vi "Connect.vi"(8 "error in (no error)":errorcluster, 9 "Custom Config Data":u8[](array[numeric]) format="%.0x", 10 "Connection Name":string, 11 "CIFTag in":refnum<class "CIF_NIChn.lvclass">) -> (0 "error out":errorcluster, 3 "CIFTag out":refnum<class "CIF_NIChn.lvclass">)   [LabVIEW 2021, in "CIF_NIChn.lvclass"]
uses:
  CIF_NIChn.lvclass
  D:/dev/CIF-LVCore/src/Channels/CIFChannels/CIFChannels.lvclass
  CIFChannels/CIFChannels.lvclass/CIFChannels.ctl
  CIFChannels/Typedef/Channel State.ctl
  CIFChannels/Accessors/Read Direction.vi
  CIFChannels/Accessors/Read Name.vi
  CIF_NIChn.lvclass/CIF_NIChn.ctl
  CIFChannels/CIFChannels.lvclass
  <vilib>/CIFChannels/CIFChannelCore.lvlib
  D:/dev/CIF-LVCore/src/Channels/CIF_NIChn/NIChn/CIF_NIChn.lvclass
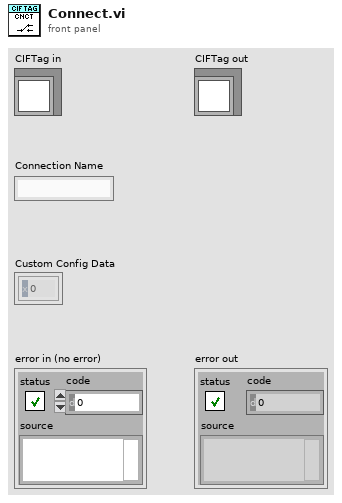
[diagram p1: front panel]
types:
  T1 = typedef "CIFChannels.lvclass/Channel State.ctl" = enum16{"Creating", "Disconnected", "Connecting", "Connected", "Destroyed"}
  T2 = typedef "CIFChannels.lvclass/Direction.ctl" = enum16{"Publisher", "Subscriber"}
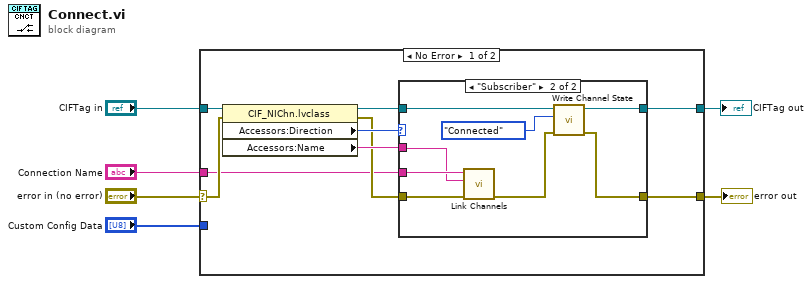
[diagram p0: block diagram]
diagram:
  n1 = case shown="No Error" "error in (no error)" {
    selector: "error in (no error)" -> [w14 w27]
    tunnel: [w7 w27] -> w5
    tunnel: [w11 w26] -> w3
    tunnel: "CIFTag in" -> [w15 w26]
    tunnel: "Connection Name" -> [w8 _]
    tunnel: "Custom Config Data" -> [_ _]
    frame No Error {
      n2 = property class="CIF_NIChn.lvclass"(reference=w15, error in=w14) -> (reference out=w13:refnum<class "CIF_NIChn.lvclass">, error out=w9:errorcluster, "Accessors:Direction"=w12:T2, "Accessors:Name"=w10:string)
      n3 = case shown="\"Subscriber\"" w12 {
        tunnel: w13 -> [w17 w25]
        tunnel: [w17 w19] -> w11
        tunnel: w10 -> [_ w23]
        tunnel: w9 -> [w16 w22]
        tunnel: w8 -> [_ w24]
        tunnel: [w16 w20] -> w7
        frame "Publisher" {
        }
        frame "Subscriber" {
          n4 = call <vilib>:"Link Channels.vi"("error in"=w22, "Consumer Channel Name"=w23, "Producer Channel Name"=w24) -> ("error out"=w21:errorcluster)  [unwired: 8 in]
          n5 = call "Write Channel State.vi"("error in (no error)"=w21, "Channel State"=Channel_State."Connected", "CIFChannels in"=w25) -> ("error out"=w20:errorcluster, "CIFChannels in"=w19:refnum<class "CIF_NIChn.lvclass">)  [unwired: 7 in]
        }
      }
    }
    frame Error {
    }
  }
  "error out" <- w5
  "CIFTag out" <- w3
